vi "ButtonAddedToControlStepperMotor_Main.vi"() -> ()   [LabVIEW 2015]
panel:
  in  "Channel 4":tag="Dev5/port0/line3"
  in  "Channel 3":tag="Dev5/port0/line2"
  in  "Channel 1":tag="Dev5/port0/line0"
  in  "Channel 2":tag="Dev5/port0/line1"
  out "error out 2":errorcluster
  out "error out":errorcluster
  in  "StepDone1":i32
  in  "Home Button":bool
  in  "Position Control":i32
  in  "Right Button":bool
  in  "Left Button":bool
  in  "Stop Button 2":bool
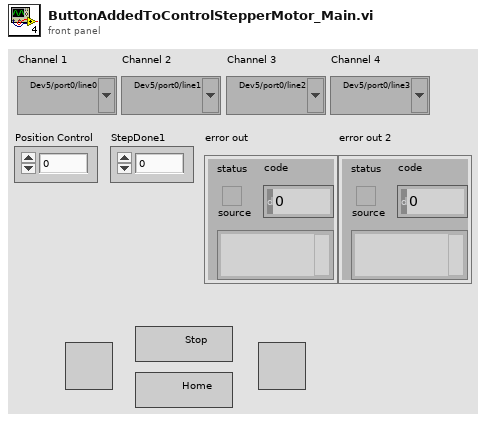
[diagram p1: front panel]
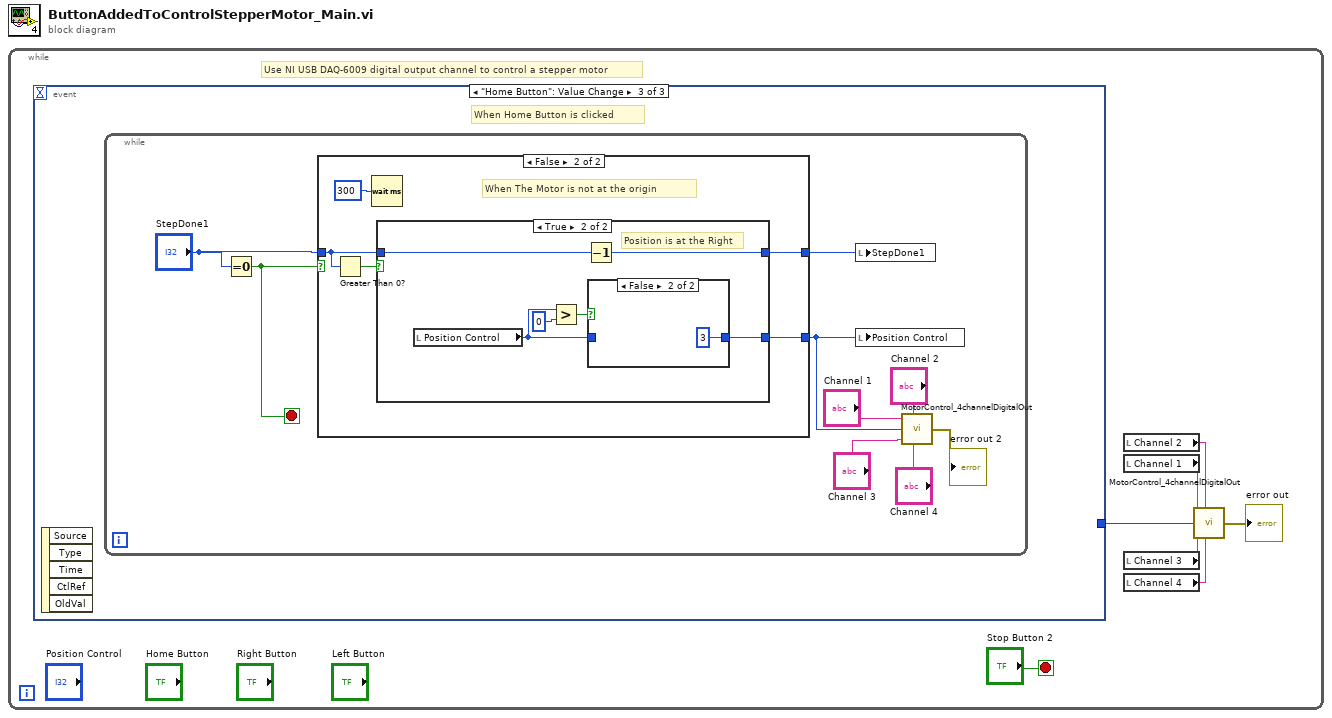
[diagram p0: block diagram]
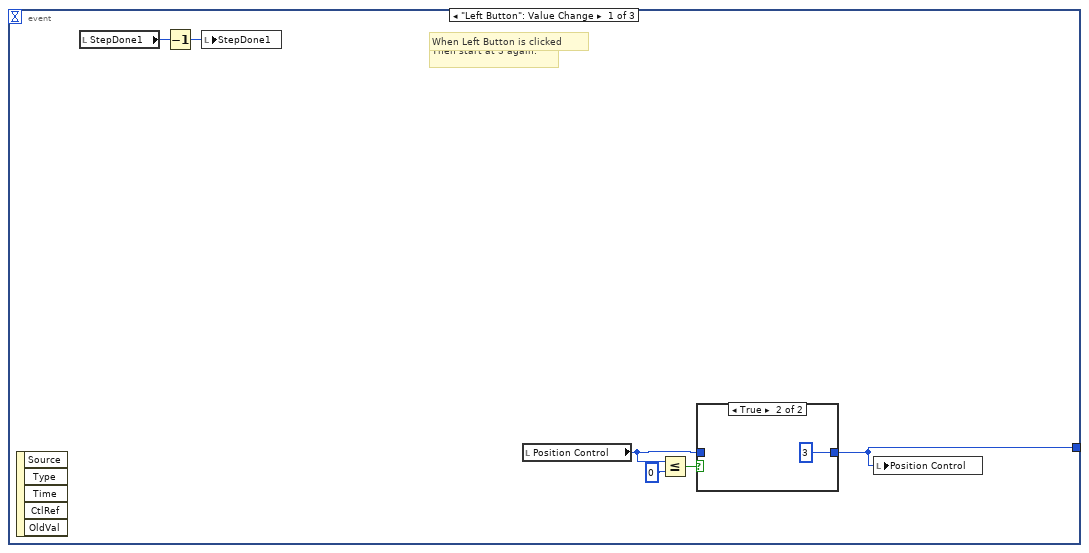
[diagram p2: hidden frame]
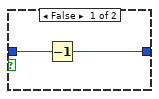
[diagram p3: hidden frame]
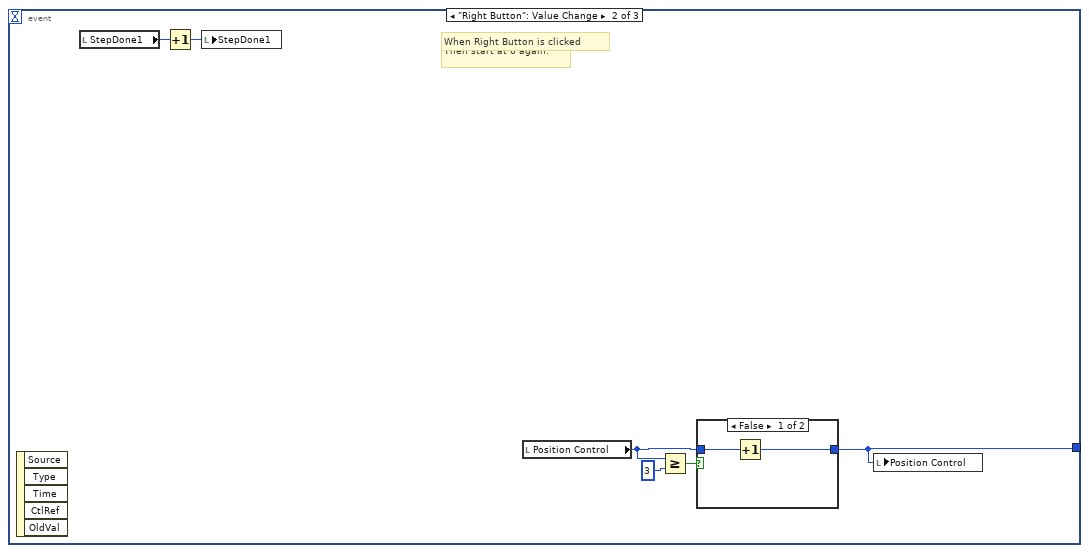
[diagram p4: hidden frame]
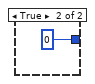
[diagram p5: hidden frame]
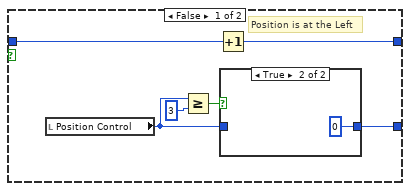
[diagram p7: hidden frame]
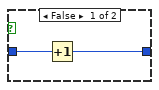
[diagram p8: hidden frame]
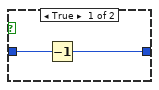
[diagram p9: hidden frame]
diagram:
  n1 = while {
    stop <- "Stop Button 2" stop-if-true
    # "Use NI USB DAQ-6009 digital output channel to control a stepper motor"
    n2 = event shown="[2] \"Home Button\": Value Change" {
      selector: _ -> [_ _ _]
      dyn-events: _ -> [_ _ _]
      timeout: _ -> [_ _ _]
      tunnel: [w8 w17 _] -> w6
      event "Left Button": Value Change {
        # "When Position is at 0.\nThen start at 3 again."
        # "When Left Button is clicked"
        n3 = event-data() -> ()  [unwired: 1 in, 5 out]
        n4 = local read "StepDone1"() -> (w9:i32)
        n5 = Decrement(x=w9) -> (x-1=w10:i32)
        n6 = local write "StepDone1"(w10) -> ()
        n7 = local read "Position Control"() -> (w11:i32)
        n8 = Less Or Equal?(x=w11, y=0) -> (x <= y?=w12:bool)
        n9 = case shown="True" w12 {
          tunnel: [w14 3 ("y")] -> w8
          tunnel: w11 -> [w15 _]
          frame False {
            n10 = Decrement(x=w15) -> (x-1=w14:i32)
          }
          frame True {
          }
        }
        n11 = local write "Position Control"(w8) -> ()
      }
      event "Right Button": Value Change {
        # "When Position is at 3.\nThen start at 0 again."
        # "When Right Button is clicked"
        n12 = event-data() -> ()  [unwired: 1 in, 5 out]
        n13 = local read "StepDone1"() -> (w19:i32)
        n14 = Increment(x=w19) -> (x+1=w18:i32)
        n15 = local write "StepDone1"(w18) -> ()
        n16 = local read "Position Control"() -> (w20:i32)
        n17 = Greater Or Equal?(x=w20, y=3) -> (x >= y?=w21:bool)
        n18 = case shown="False" w21 {
          tunnel: [w23 0 ("y")] -> w17
          tunnel: w20 -> [w24 _]
          frame False {
            n19 = Increment(x=w24) -> (x+1=w23:i32)
          }
          frame True {
          }
        }
        n20 = local write "Position Control"(w17) -> ()
      }
      event "Home Button": Value Change {
        # "When Home Button is clicked"
        n21 = event-data() -> ()  [unwired: 1 in, 5 out]
        n22 = while {
          stop <- w26 stop-if-true
          n23 = Equal To 0?(x="StepDone1") -> (x = 0?=w26:bool)
          n24 = case shown="False" w26 {
            tunnel: "StepDone1" -> [w35 w37]
            tunnel: [w35 w39] -> w33
            tunnel: [_ w38] -> w32
            frame True {
              # "When The Motor is at the origin"
            }
            frame False {
              # "When The Motor is not at the origin"
              n25 = Greater Than 0?(x=w37) -> (x > 0?=w40:bool)
              n26 = Wait (ms)(milliseconds to wait=u32 300) -> ()  [unwired: 1 out]
              n27 = case shown="True" w40 {
                tunnel: [w44 w53] -> w39
                tunnel: [w43 w52] -> w38
                tunnel: w37 -> [w41 w50]
                frame False {
                  # "Position is at the Left"
                  n28 = local read "Position Control"() -> (w42:i32)
                  n29 = Greater Or Equal?(x=w42, y=3) -> (x >= y?=w46:bool)
                  n30 = Increment(x=w41) -> (x+1=w44:i32)
                  n31 = case shown="True" w46 {
                    tunnel: [w48 0 ("y")] -> w43
                    tunnel: w42 -> [w47 _]
                    frame False {
                      n32 = Increment(x=w47) -> (x+1=w48:i32)
                    }
                    frame True {
                    }
                  }
                }
                frame True {
                  # "Position is at the Right"
                  n33 = local read "Position Control"() -> (w51:i32)
                  n34 = Greater?(x=w51, y=0) -> (0:w54:bool)
                  n35 = Decrement(x=w50) -> (x-1=w53:i32)
                  n36 = case shown="False" w54 {
                    tunnel: [w56 3 ("y")] -> w52
                    tunnel: w51 -> [w57 _]
                    frame True {
                      n37 = Decrement(x=w57) -> (x-1=w56:i32)
                    }
                    frame False {
                    }
                  }
                }
              }
            }
          }
          n38 = local write "StepDone1"(w33) -> ()
          n39 = local write "Position Control"(w32) -> ()
          n40 = call "MotorControl_4channelDigitalOut.vi"("Channel 1"="Channel 1", "Channel 2"="Channel 2", "Motor Position Control"=w32, "Channel 3"="Channel 3", "Channel 4"="Channel 4") -> ("error out"=→"error out 2":errorcluster)
        }
      }
    }
    n41 = local read "Channel 2"() -> (w3:tag)
    n42 = local read "Channel 1"() -> (w4:tag)
    n43 = local read "Channel 3"() -> (w2:tag)
    n44 = local read "Channel 4"() -> (w1:tag)
    n45 = call "MotorControl_4channelDigitalOut.vi"("Channel 1"=w4, "Channel 2"=w3, "Motor Position Control"=w6, "Channel 3"=w2, "Channel 4"=w1) -> ("error out"=→"error out":errorcluster)
  }
